vi "Run Pre-Variable Hook.vi"(8 "Error In":errorcluster, 10 "Tag In":refnum<class "Variable.lvclass">, 11 "Renderer In":refnum<class "Renderer.lvclass">) -> (0 "Error Out":errorcluster, 2 "Tag Out":refnum<class "Variable.lvclass">, 3 "Renderer Out":refnum<class "Renderer.lvclass">)   [LabVIEW 2018, in "Toolkit.lvlib" / "Renderer.lvclass"]
uses:
  Renderer.lvclass
  Nodes/Variable/Variable.lvclass
  Renderer.lvclass/Renderer.ctl
  Hooks/Render/Variable/Variable.lvclass
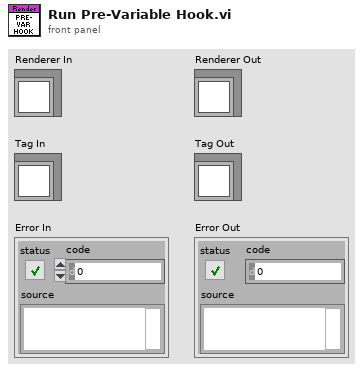
[diagram p1: front panel]
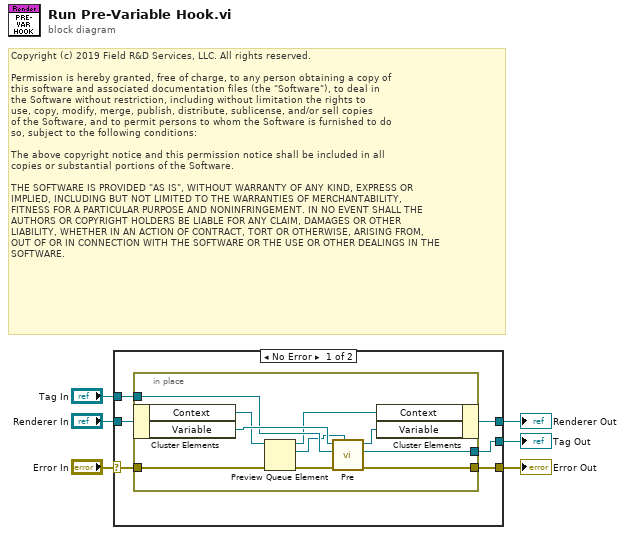
[diagram p0: block diagram]
diagram:
  # "Copyright (c) 2019 Field R&D Services, LLC. All rights reserved.\n\nPermission is hereby granted, free of charge, to any person obtaining a copy of\nthis software and associated documentation files (the \"Software\"), to deal in\nthe Software without restriction, including without limitation the rights to\nuse, copy, modify, merge, publish, distribute, sublicense, and/or sell copies\nof the Software, and to permit persons to whom the Software is furnished to do\nso, subject to the following conditions:\n\nThe above copyright notice and this permission notice shall be included in all\ncopies or substantial portions of the Software.\n\nTHE SOFTWARE IS PROVIDED \"AS IS\", WITHOUT WARRANTY OF ANY KIND, EXPRESS OR\nIMPLIED, INCLUDING BUT NOT LIMITED TO THE WARRANTIES OF MERCHANTABILITY,\nFITNESS FOR A PARTICULAR PURPOSE AND NONINFRINGEMENT. IN NO EVENT SHALL THE\nAUTHORS OR COPYRIGHT HOLDERS BE LIABLE FOR ANY CLAIM, DAMAGES OR OTHER\nLIABILITY, WHETHER IN AN ACTION OF CONTRACT, TORT OR OTHERWISE, ARISING FROM,\nOUT OF OR IN CONNECTION WITH THE SOFTWARE OR THE USE OR OTHER DEALINGS IN THE\nSOFTWARE."
  n1 = case shown="No Error" "Error In" {
    selector: "Error In" -> [w12 w24]
    tunnel: "Renderer In" -> [w9 w25]
    tunnel: [w11 w25] -> w1
    tunnel: [w10 w24] -> w5
    tunnel: "Tag In" -> [w8 w23]
    tunnel: [w7 w23] -> w3
    frame No Error {
      n2 = in-place {
        in-place-border: w12 -> [w15]
        in-place-border: [w20] -> w10
        in-place-border: w8 -> [w19]
        in-place-border: [w18] -> w7
        n3 = in-place-cluster #1(w9) -> ("Context"=w17:refnum<queue>, "Variable"=w22:refnum<class "Variable.lvclass">)
        n4 = Preview Queue Element(queue=w17, error in (no error)=w15) -> (queue out=w16:refnum<queue>, element=w13:refnum<class "Datum.lvclass">, error out=w14:errorcluster)  [unwired: 1 in, 1 out]
        n5 = call-dynamic "Pre.vi"("Datum"=w13, "Error In"=w14, "Tag In"=w19, "Render Variable In"=w22) -> ("Error Out"=w20:errorcluster, "Tag Out"=w18:refnum<class "Variable.lvclass">, "Render Variable Out"=w21:refnum<class "Variable.lvclass">)  [unwired: 5 in]
        n6 = in-place-cluster #1("Context"=w16, "Variable"=w21) -> (w11:refnum<class "Renderer.lvclass">)
      }
    }
    frame Error {
    }
  }
  "Error Out" <- w5
  "Tag Out" <- w3
  "Renderer Out" <- w1
